vi "外观 1.vi"(0 "Data In":T4 caption="数据输入", 2 "Display State In":T2 caption="显示状态输入", 3 "Container State":T3 caption="容器状态") -> (6 "Data Out":T4 caption="数据输出", 7 "Display State Out":T2 caption="显示状态输出", 8 "Action":T1 caption="动作")   [LabVIEW 2016, in "多参数状态显示.xctl"]
uses:
  <vilib>/_xctls/Container State.ctl
  <vilib>/_xctls/Action.ctl
  <vilib>/_xctls/XControlSupport.lvlib
panel:
  out "数据标识":string="N"
  out "状态2":string="7.87 mg/L"
  out "状态1":string="78.56 %"
  out "标签名":string="水温"
  out "标签底板":string
  out "检测值2趋势":dbl
  out "检测值1趋势":dbl
  out "标签底板 2":string
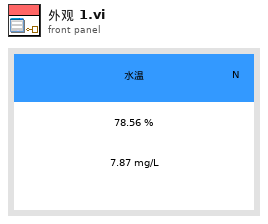
[diagram p1: front panel]
types:
  T1 = typedef "XControlSupport.lvlib/Action.ctl" = cluster{"Data Changed?":bool, "State Changed?":bool, "Action Name":string}
  T2 = typedef "多参数状态显示.xctl/状态 1.ctl" = cluster{"数值":dbl}
  T3 = typedef "XControlSupport.lvlib/Container State.ctl" = cluster{"Indicator?":bool, "Run Mode?":bool, " Refnum":refnum<vi>}
  T4 = typedef "多参数状态显示.xctl/数据 1.ctl" = cluster{"标签":string, "检测值1":cluster{"检测值":dbl, "单位":string, "启用":bool}, "检测值2":cluster{"检测值":dbl, "单位":string, "启用":bool}, "数据标识":string}
  T5 = typedef "LVPoint32TypeDef.ctl" = cluster{"Horizontal":i32, "Vertical":i32}
  T6 = typedef "LVRectTypeDef.ctl" = cluster{"Left":i16, "Top":i16, "Right":i16, "Bottom":i16}
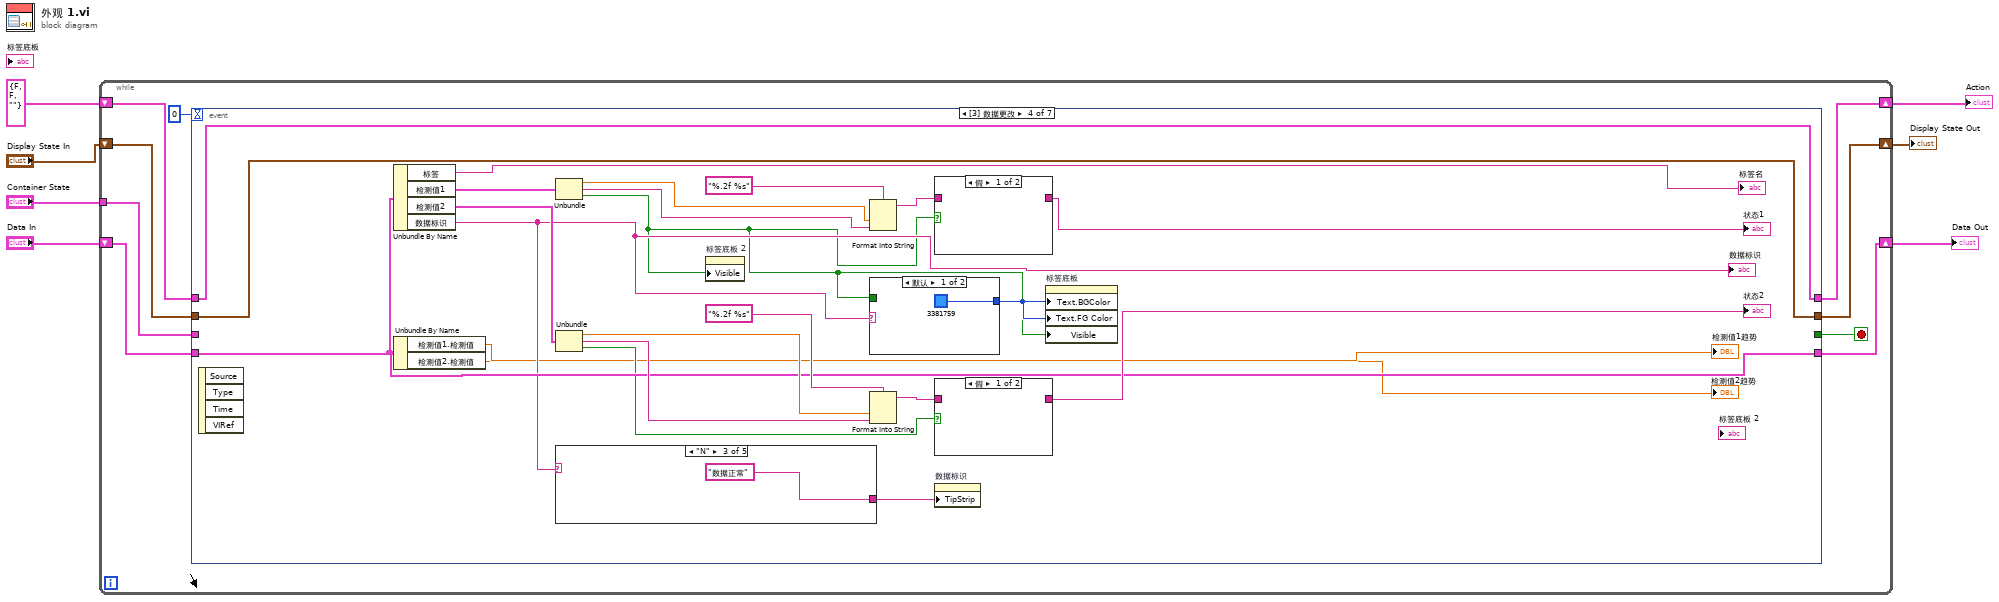
[diagram p0: block diagram]
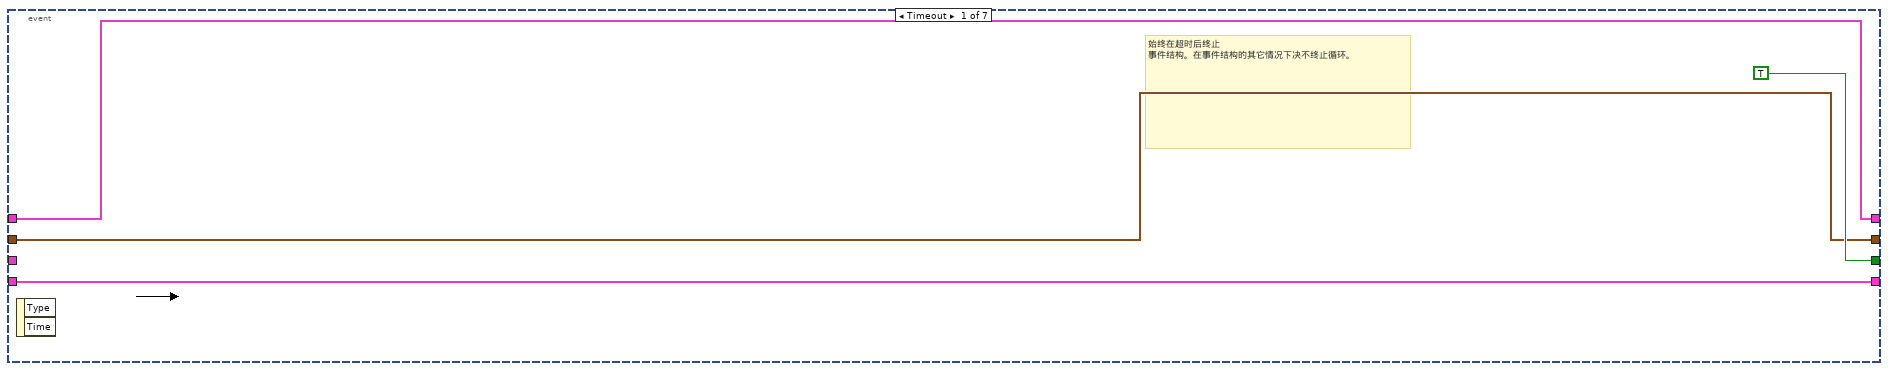
[diagram p2: hidden frame]
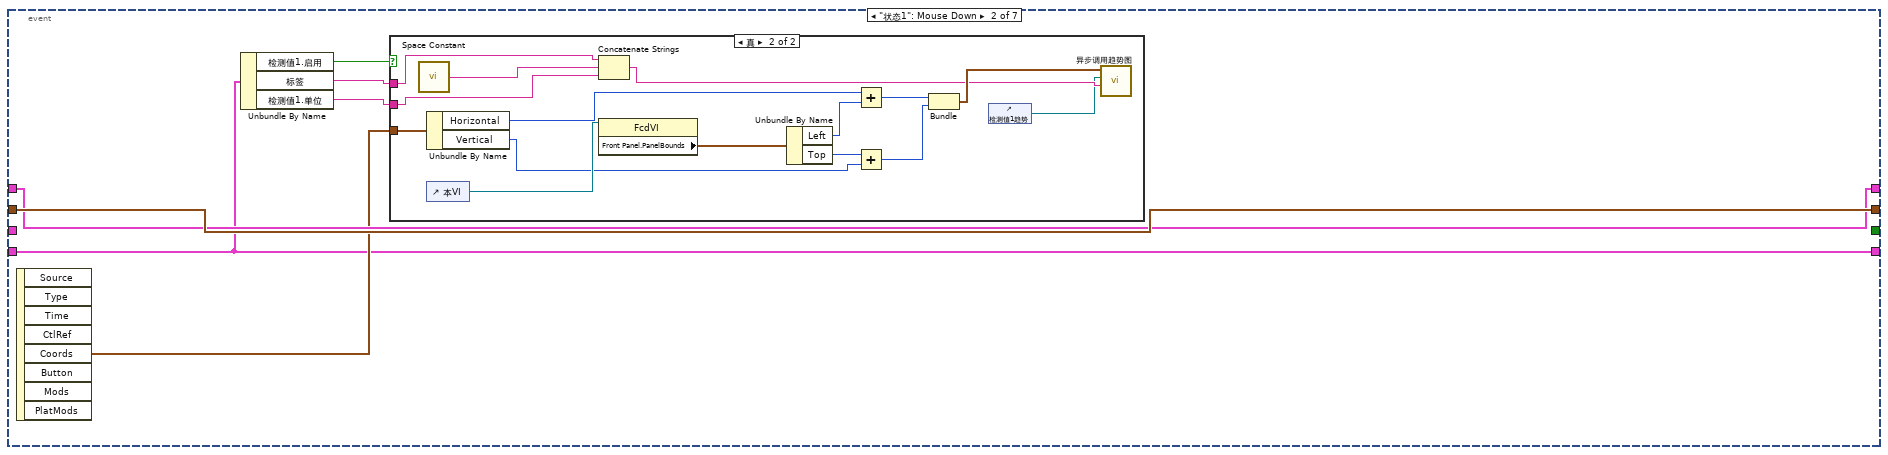
[diagram p3: hidden frame]
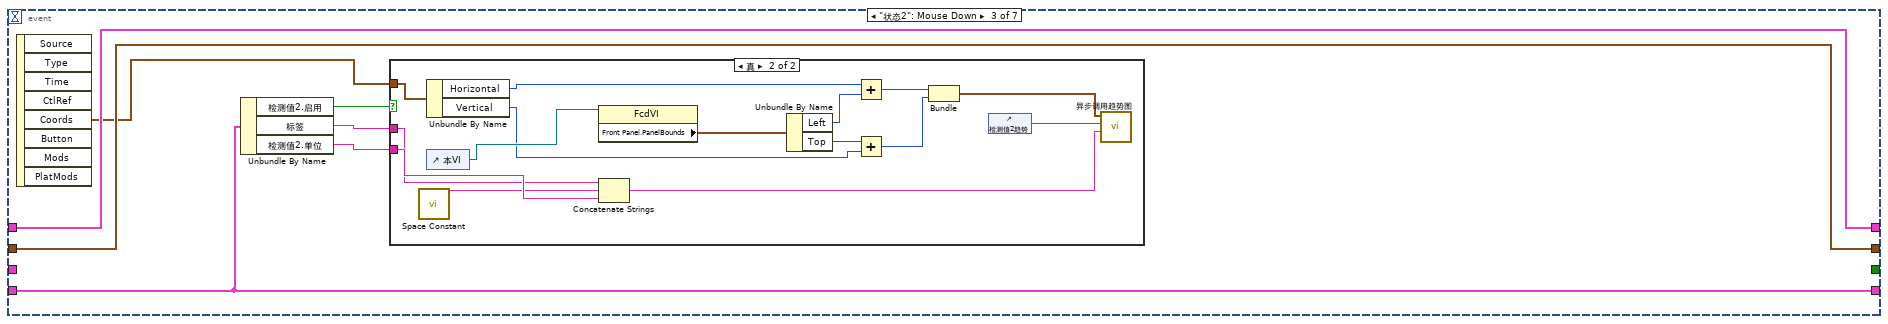
[diagram p5: hidden frame]
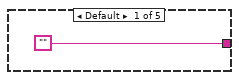
[diagram p7: hidden frame]
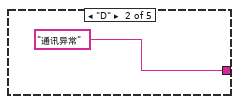
[diagram p8: hidden frame]
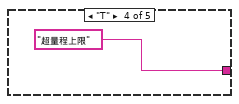
[diagram p9: hidden frame]
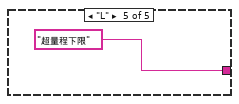
[diagram p10: hidden frame]
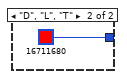
[diagram p13: hidden frame]
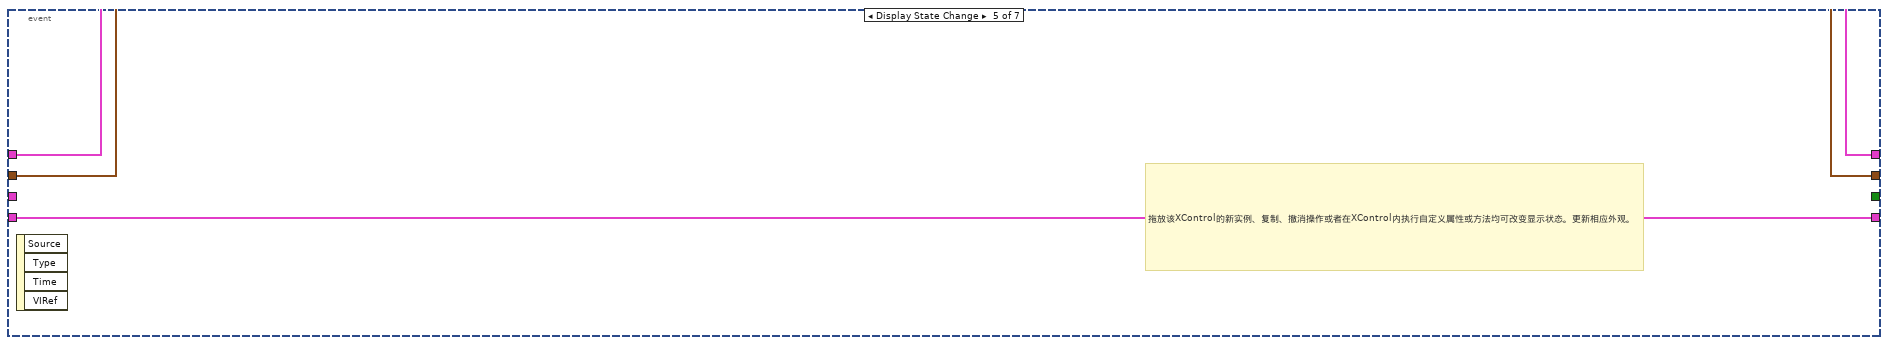
[diagram p14: hidden frame]
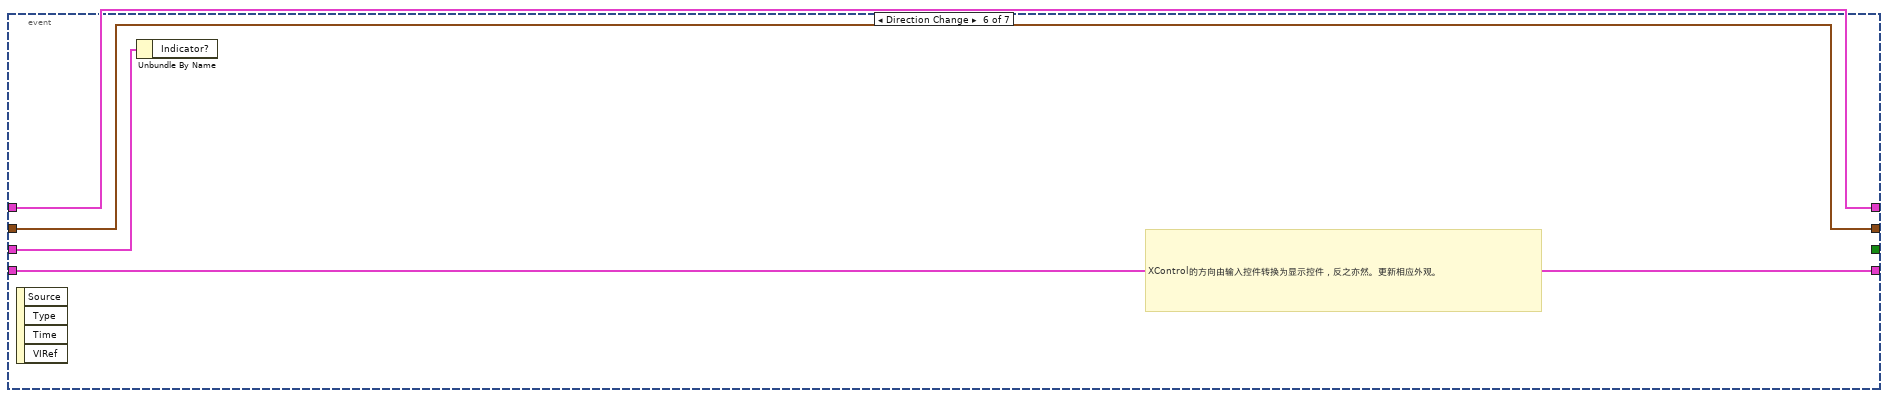
[diagram p15: hidden frame]
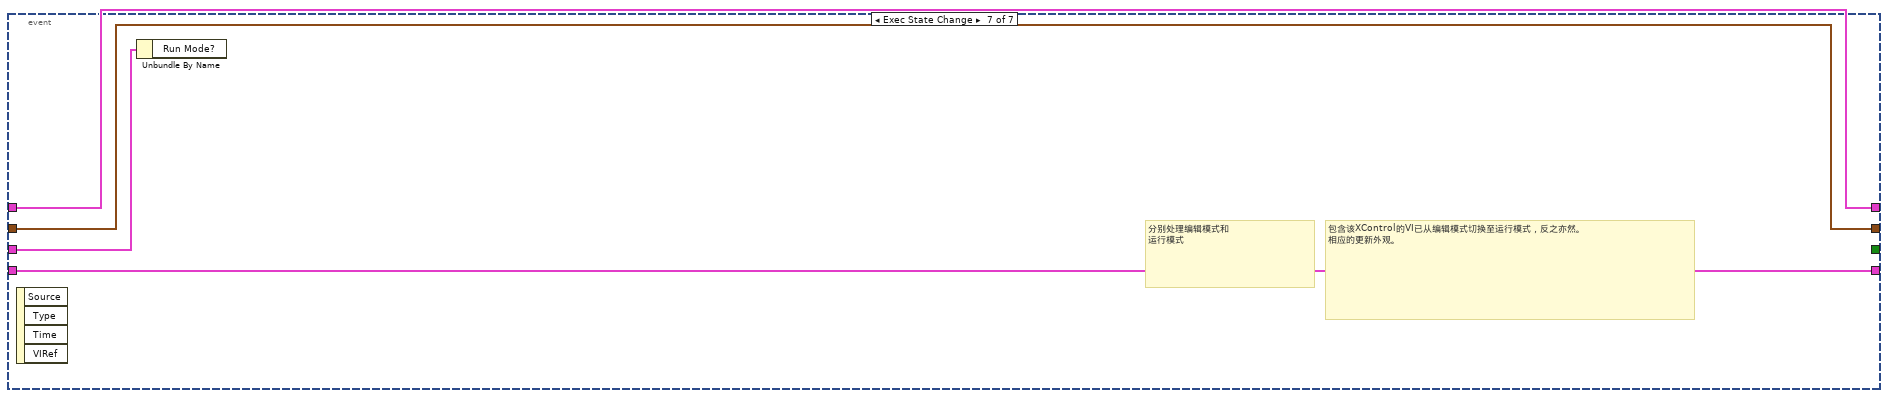
[diagram p16: hidden frame]
diagram:
  n1 = while {
    shift-right: [w15] -> w4
    shift-left: "Display State In" -> [w16]
    tunnel: "Container State" -> [w12]
    shift-right: [w10] -> w7
    shift-left: "Data In" -> [w11]
    shift-right: [w8] -> w2
    shift-left: T1 {"Data Changed?"=FALSE, "State Changed?"=FALSE, "Action Name"=""} ("Action") -> [w9]
    stop <- w14 stop-if-true
    n2 = event shown="[3] 数据更改" {
      selector: _ -> [_ _ _ _ _ _ _]
      dyn-events: _ -> [_ _ _ _ _ _ _]
      timeout: 0 -> [_ _ _ _ _ _ _]
      tunnel: w16 -> [w18 w27 w49 w87 w97 w102 w106]
      tunnel: [w18 w27 w49 w87 w97 w102 w106] -> w15
      tunnel: [TRUE _ _ _ _ _ _] -> w14
      tunnel: w12 -> [_ _ _ _ _ w103 w107]
      tunnel: w11 -> [w17 w24 w46 w72 w99 w101 w105]
      tunnel: [w17 w24 w46 w72 w99 w101 w105] -> w10
      tunnel: [w19 w26 w48 w86 w98 w100 w104] -> w8
      tunnel: w9 -> [w19 w26 w48 w86 w98 w100 w104]
      event Timeout {
        # "始终在超时后终止\n事件结构。在事件结构的其它情况下决不终止循环。"
        n3 = event-data() -> ()  [unwired: 1 in, 2 out]
      }
      event "状态1": Mouse Down {
        n4 = event-data() -> ("Coords"=w25:T5)  [unwired: 1 in, 7 out]
        n5 = Unbundle By Name(w24) -> ("检测值1.启用"=w23:bool, "标签"=w22:string, "检测值1.单位"=w21:string)
        n6 = case shown="真" w23 {
          tunnel: w25 -> [_ w39]
          tunnel: w22 -> [_ w32]
          tunnel: w21 -> [_ w31]
          frame False {
          }
          frame True {
            n7 = call <vilib>:"Space Constant.vi"() -> ("String"=w29:string)
            n8 = Unbundle By Name(w39) -> ("Horizontal"=w38:i32, "Vertical"=w36:i32)
            n9 = control-ref of="本VI"() -> (w42:refnum<vi>)
            n10 = Concatenate Strings(w32, w29, w31) -> (w30:string)
            n11 = property class="FcdVI"(reference=w42) -> ("Front Panel.PanelBounds"=w40:T6)  [unwired: 1 in, 2 out]
            n12 = Unbundle By Name(w40) -> ("Left"=w41:i16, "Top"=w37:i16)
            n13 = Add(x=w38, y=w41) -> (x+y=w35:i32)
            n14 = Add(x=w37, y=w36) -> (x+y=w34:i32)
            n15 = Bundle(w35, w34) -> (w33:cluster{i32, i32})  [unwired: 1 in]
            n16 = control-ref of="检测值1趋势"() -> (w28:refnum<vi>)
            n17 = call "异步调用趋势图.vi"("参数"=w30, "Array输入"=w28, "原点"=w33) -> ()  [unwired: 9 in]
          }
        }
      }
      event "状态2": Mouse Down {
        n18 = event-data() -> ("Coords"=w47:T5)  [unwired: 1 in, 7 out]
        n19 = Unbundle By Name(w46) -> ("检测值2.启用"=w45:bool, "标签"=w44:string, "检测值2.单位"=w43:string)
        n20 = case shown="真" w45 {
          tunnel: w47 -> [_ w61]
          tunnel: w44 -> [_ w52]
          tunnel: w43 -> [_ w54]
          frame False {
          }
          frame True {
            n21 = call <vilib>:"Space Constant.vi"() -> ("String"=w51:string)
            n22 = Unbundle By Name(w61) -> ("Horizontal"=w60:i32, "Vertical"=w58:i32)
            n23 = control-ref of="本VI"() -> (w64:refnum<vi>)
            n24 = property class="FcdVI"(reference=w64) -> ("Front Panel.PanelBounds"=w62:T6)  [unwired: 1 in, 2 out]
            n25 = Concatenate Strings(w52, w51, w54) -> (w53:string)
            n26 = Unbundle By Name(w62) -> ("Left"=w63:i16, "Top"=w59:i16)
            n27 = Add(x=w60, y=w63) -> (x+y=w57:i32)
            n28 = Add(x=w59, y=w58) -> (x+y=w56:i32)
            n29 = Bundle(w57, w56) -> (w55:cluster{i32, i32})  [unwired: 1 in]
            n30 = control-ref of="检测值2趋势"() -> (w50:refnum<vi>)
            n31 = call "异步调用趋势图.vi"("参数"=w53, "Array输入"=w50, "原点"=w55) -> ()  [unwired: 9 in]
          }
        }
      }
      event Data Change {
        n32 = event-data() -> ()  [unwired: 1 in, 4 out]
        n33 = Unbundle By Name(w72) -> ("标签"=→"标签名":string, "检测值1"=w84:cluster{"检测值":dbl, "单位":string, "启用":bool}, "检测值2"=w77:cluster{"检测值":dbl, "单位":string, "启用":bool}, "数据标识"=w69:string)
        "数据标识" <- w69
        n34 = Unbundle By Name(w72) -> ("检测值1.检测值"=→"检测值1趋势":dbl, "检测值2.检测值"=→"检测值2趋势":dbl)
        n35 = Unbundle(w84) -> ("检测值"=w83:dbl, "单位"=w82:string, "启用"=w67:bool)
        n36 = Unbundle(w77) -> ("检测值"=w78:dbl, "单位"=w79:string, "启用"=w71:bool)
        n37 = case shown="\"N\"" w69 {
          tunnel: ["" "通讯异常" "数据正常" "超量程上限" "超量程下限"] -> w68
          frame Default {
          }
          frame "D" {
          }
          frame "N" {
          }
          frame "T" {
          }
          frame "L" {
          }
        }
        n38 = property on="标签底板 2" class="Str"("Visible"=w67) -> ()  [unwired: 2 in, 2 out]
        n39 = Format Into String(format string="%.2f %s" ("格式字符串"), w83, w82) -> (resulting string=w74:string)  [unwired: 2 in, 1 out]
        n40 = case shown="默认" w69 {
          tunnel: [u32 3381759 u32 16711680] -> w70
          tunnel: w67 -> [_ _]
          frame Default {
          }
          frame "D", "L", "T" {
          }
        }
        n41 = Format Into String(format string="%.2f %s" ("格式字符串"), w78, w79) -> (resulting string=w75:string)  [unwired: 2 in, 1 out]
        n42 = case shown="假" w67 {
          tunnel: [_ w93] -> w73
          tunnel: w74 -> [_ w93]
          frame False {
          }
          frame True {
          }
        }
        "状态1" <- w73
        n43 = case shown="假" w71 {
          tunnel: [_ w94] -> w76
          tunnel: w75 -> [_ w94]
          frame False {
          }
          frame True {
          }
        }
        "状态2" <- w76
        n44 = property on="数据标识" class="Str"("TipStrip"=w68) -> ()  [unwired: 2 in, 2 out]
        n45 = property on="标签底板" class="Str"("Text.BGColor"=w70, "Text.FG Color"=w70, "Visible"=w67) -> ()  [unwired: 2 in, 2 out]
      }
      event Display State Change {
        # "拖放该XControl的新实例、复制、撤消操作或者在XControl内执行自定义属性或方法均可改变显示状态。更新相应外观。"
        n46 = event-data() -> ()  [unwired: 1 in, 4 out]
      }
      event Direction Change {
        # "XControl的方向由输入控件转换为显示控件，反之亦然。更新相应外观。"
        n47 = event-data() -> ()  [unwired: 1 in, 4 out]
        n48 = Unbundle By Name(w103) -> ()  [unwired: 1 out]
      }
      event Exec State Change {
        # "包含该XControl的VI已从编辑模式切换至运行模式，反之亦然。\n相应的更新外观。"
        # "分别处理编辑模式和\n运行模式"
        n49 = event-data() -> ()  [unwired: 1 in, 4 out]
        n50 = Unbundle By Name(w107) -> ()  [unwired: 1 out]
      }
    }
  }
  "Display State Out" <- w4
  "Data Out" <- w7
  "Action" <- w2
